vi "Button 2.vi"(8 "error in (no error)":errorcluster, 11 "button value":bool) -> (0 "error out":errorcluster)   [LabVIEW 2014]
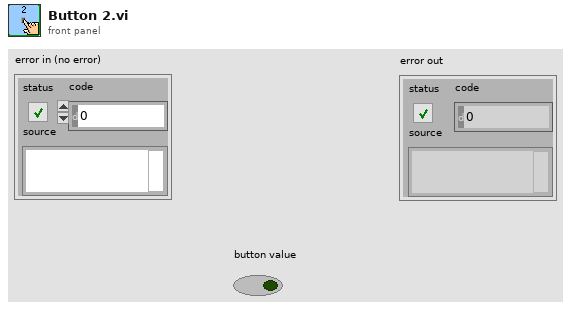
[diagram p1: front panel]
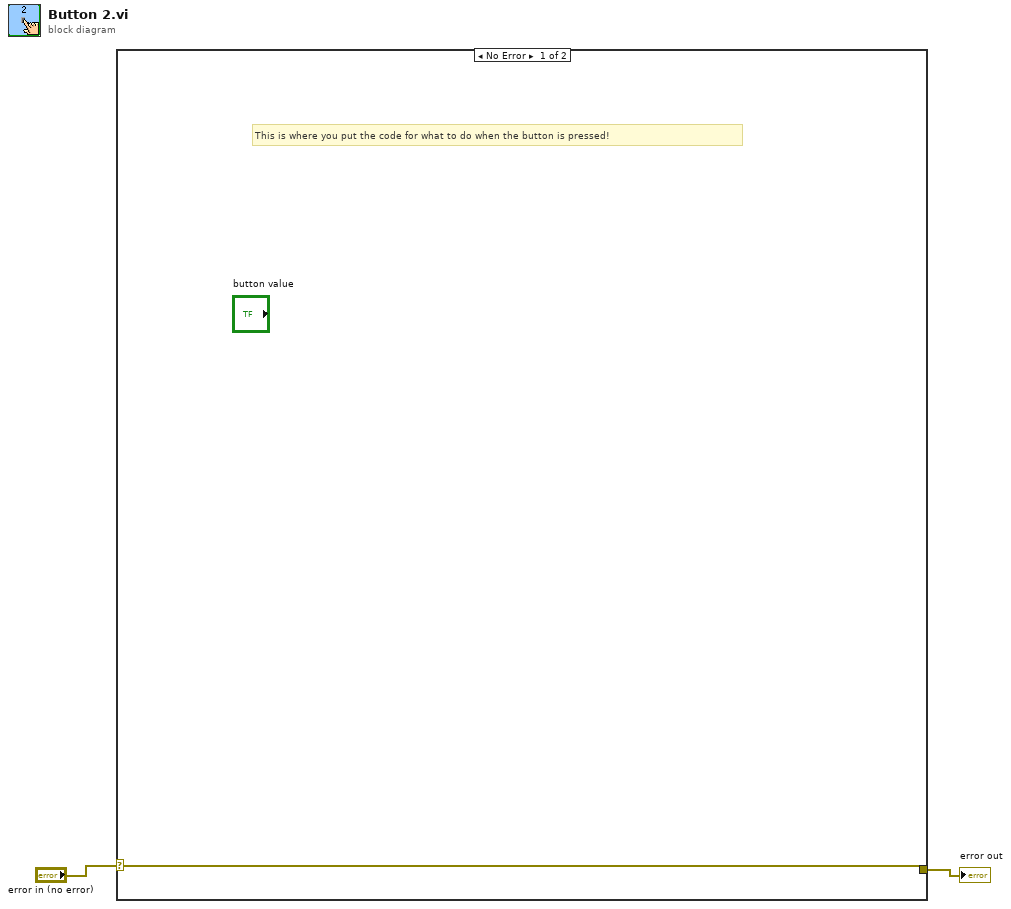
[diagram p0: block diagram]
diagram:
  n1 = case shown="No Error" "error in (no error)" {
    selector: "error in (no error)" -> [w3 w4]
    tunnel: [w3 w4] -> w1
    frame No Error {
      # "This is where you put the code for what to do when the button is pressed!"
    }
    frame Error {
      # "This is what to do if there is an error.  Usually it is nothing."
    }
  }
  "error out" <- w1
